vi "Check ToStim Queue.vi"(8 "error in (no error)":errorcluster, 11 "Stim Player Data In":T1) -> (0 "error out":errorcluster, 3 "Stim Player Data Out":T1, 4 "Error?":bool)   [LabVIEW 2011]
uses:
  Controls/Stim Player Data.ctl
  Controls/Top Level Control.ctl
  <vilib>/NI/AMC/Message Queue.ctl
  <vilib>/NI/AMC/Message.ctl
  <vilib>/NI/Tools/Keyed Array/KeyedArray.ctl
  Controls/ListBox Test Record.ctl
  Controls/DVR of CSV Tests Data.ctl
  Controls/CSVs Tests Data.ctl
  Controls/Test Column Data.ctl
  Controls/Options DVR.ctl
  Controls/Options.ctl
  <vilib>/NI Veristand/Execution/Workspace/WorkspaceAPI.ctl
  NationalInstruments.VeriStand.ClientAPI
  <vilib>/NI Veristand/Execution/SequenceExecutionInterface/Stimulus Profile Session Ref.ctl
  <vilib>/NI Veristand/Execution/ChannelFaultManager/ChannelFaultAPI.ctl
  <vilib>/NI/AMC/Create Single Message.vi
  <vilib>/NI/AMC/Update Message Routing Info.vi
  <vilib>/NI/AMC/Read Termination Message.vi
  <vilib>/NI/AMC/Globals.vi
  <vilib>/NI/AMC/Send Message.vi
  <vilib>/NI Veristand/Execution/SequenceExecutionInterface/NI_VS Sequence Execution Interface.lvlib
  <vilib>/NI/AMC/AMC.lvlib
  <vilib>/NI/Tools/Keyed Array/Tools_KeyedArray.lvlib
  <vilib>/NI Veristand/Execution/Workspace/NI_VS Workspace ExecutionAPI.lvlib
  <vilib>/NI Veristand/Execution/ChannelFaultManager/NI_VS ChannelFault ExecutionAPI.lvlib
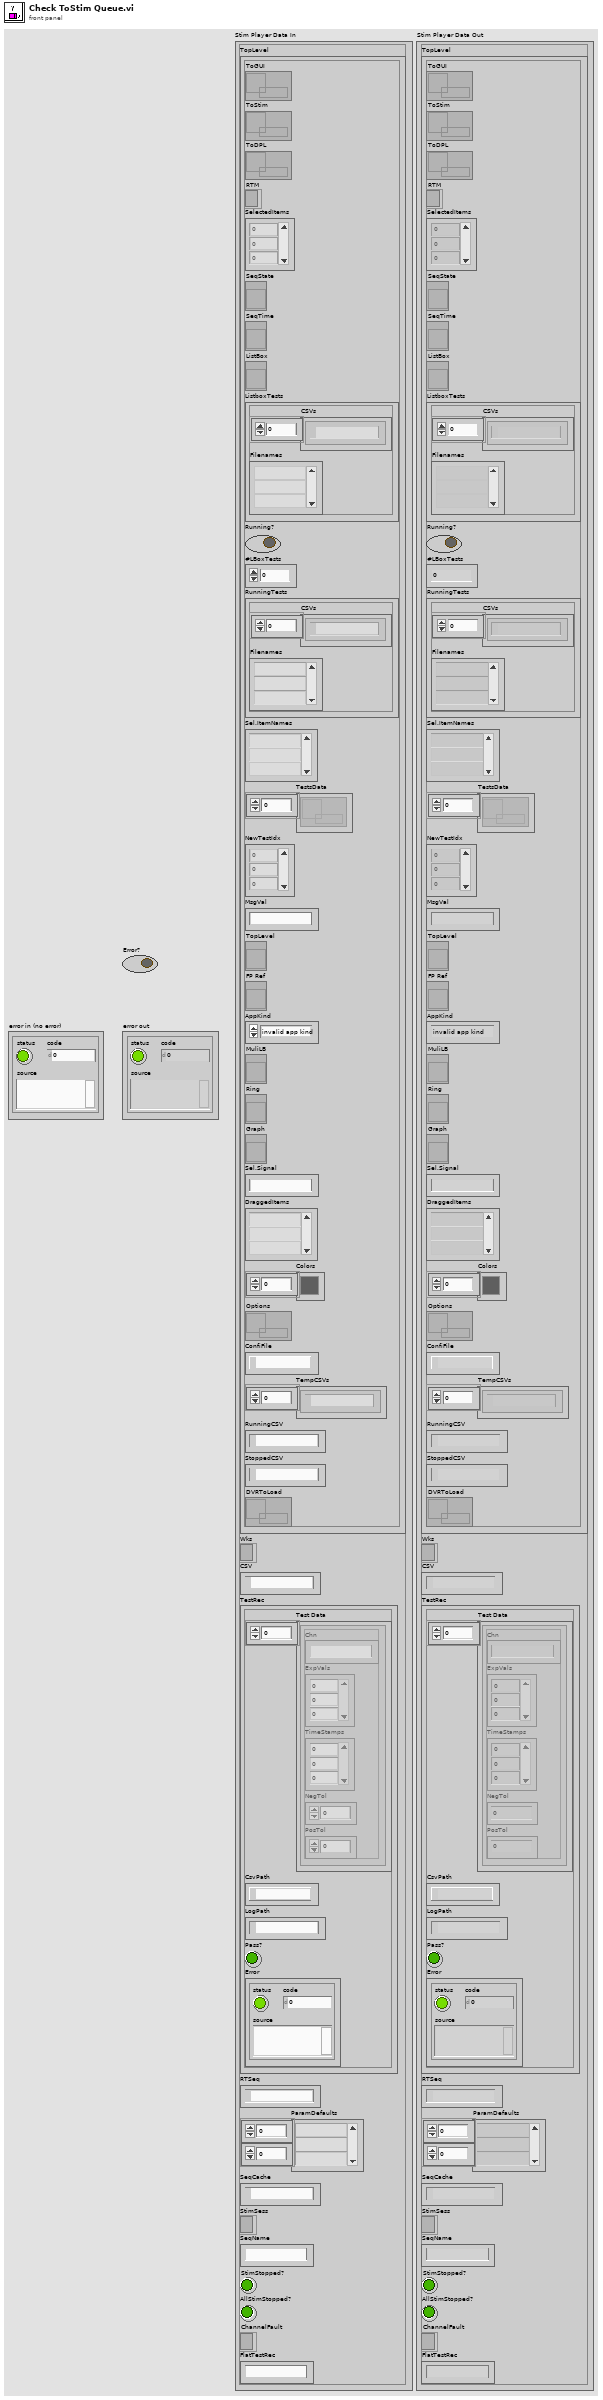
[diagram p1: front panel]
types:
  T1 = typedef "Stim Player Data.ctl" = cluster{"TopLevel":T2, "Wks":T7, "CSV":path, "TestRec":T8, "RTSeq":path, "ParamDefaults":string[][], "SeqCache":path, "StimSess":T10, "SeqName":string, "StimStopped?":bool, "AllStimStopped?":bool, "ChannelFault":T11, "FlatTestRec":string}
  T2 = typedef "Top Level Control.ctl" = cluster{"ToGUI":T3, "ToStim":T3, "ToDPL":T3, "RTM":refnum<k9>, "SelectedItems":i32[], "SeqState":refnum<vi>, "SeqTime":refnum<vi>, "ListBox":refnum<vi>, "ListboxTests":T4, "Running?":bool, "#LBoxTests":i32, "RunningTests":T4, "Sel.ItemNames":string[], "TestsData":T5[], "NewTestIdx":i32[], "MsgVal":string, "TopLevel":refnum<vi>, "FP Ref":refnum<vi>, "AppKind":enum32{"invalid app kind", "Development System", "Run Time System", "Student Edition", "Embedded LabVIEW", "Evaluation", "Custom"}, "MuliLB":refnum<vi>, "Ring":refnum<vi>, "Graph":refnum<vi>, "Sel.Signal":string, "DraggedItems":string[], "Colors":u32[], "Options":T6, "ConfiFile":path, "TempCSVs":path[], "RunningCSV":path, "StoppedCSV":path, "DVRToLoad":T5}
  T3 = typedef "AMC.lvlib/Message Queue.ctl" = refnum<queue>
  T4 = typedef "ListBox Test Record.ctl" = cluster{"CSVs":path[], "Filenames":string[]}
  T5 = typedef "DVR of CSV Tests Data.ctl" = refnum<data-value>
  T6 = typedef "Options DVR.ctl" = refnum<data-value>
  T7 = typedef "NI_VS Workspace ExecutionAPI.lvlib/WorkspaceAPI.ctl" = refnum<k24>
  T8 = typedef "CSVs Tests Data.ctl" = cluster{"Test Data":T9[], "CsvPath":path, "LogPath":path, "Pass?":bool, "Error":errorcluster}
  T9 = typedef "Test Column Data.ctl" = cluster{"Chn":string, "ExpVals":dbl[], "TimeStamps":i64[], "NegTol":dbl, "PosTol":dbl}
  T10 = typedef "NI_VS Sequence Execution Interface.lvlib/Stimulus Profile Session Ref.ctl" = refnum<k24>
  T11 = typedef "NI_VS ChannelFault ExecutionAPI.lvlib/ChannelFaultAPI.ctl" = refnum<k24>
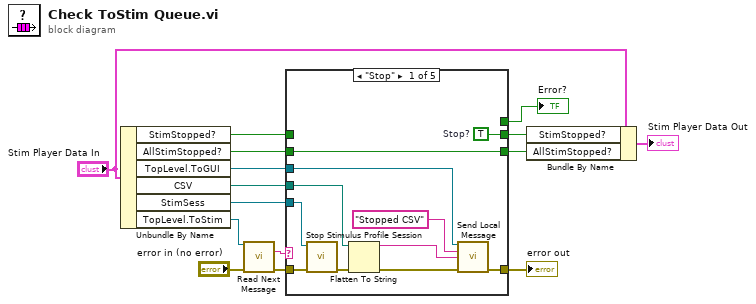
[diagram p0: block diagram]
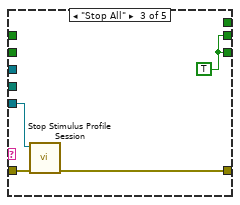
[diagram p3: hidden frame]
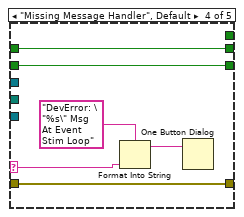
[diagram p4: hidden frame]
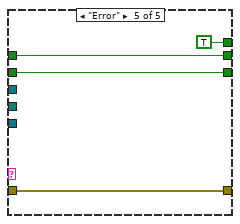
[diagram p5: hidden frame]
diagram:
  n1 = Unbundle By Name("Stim Player Data In") -> ("StimStopped?"=w10:bool, "AllStimStopped?"=w9:bool, "TopLevel.ToGUI"=w2:T3, "CSV"=w1:path, "StimSess"=w3:T10, "TopLevel.ToStim"=w4:T3)
  n2 = call <vilib>:"Read Next Message.vi"("message queue in"=w4, "error in"="error in (no error)") -> ("message name"=w11:string, "error out"=w12:errorcluster)  [unwired: 6 in, 6 out]
  n3 = case shown="\"Stop\"" w11 {
    selector: w11 -> [_ _ _ w37 _]
    tunnel: w12 -> [w26 w29 w33 w36 w43]
    tunnel: [w25 w29 w32 w36 w43] -> w14
    tunnel: [_ _ _ _ TRUE] -> w15
    tunnel: w9 -> [w20 w28 _ w35 w42]
    tunnel: [w20 w28 w31 w35 w42] -> w5
    tunnel: w10 -> [_ w27 _ w34 w40]
    tunnel: [w19 w27 w31 w34 w40] -> w6
    tunnel: w3 -> [w18 _ w30 _ _]
    tunnel: w2 -> [w17 _ _ _ _]
    tunnel: w1 -> [w16 _ _ _ _]
    frame "Stop" {
      w19 = TRUE  # Stop?
      n4 = call <vilib>:"Stop Stimulus Profile Session.vi"("error in (no error)"=w26, "Session Ref in"=w18) -> ("error out"=w24:errorcluster)  [unwired: 8 in, 1 out]
      n5 = Flatten To String(anything=w16, error in (no error)=w24) -> (data string=w22:string, error out=w21:errorcluster)  [unwired: 2 in, 1 out]
      n6 = call <vilib>:"Send Local Message.vi"("message queue in"=w17, "message name"="Stopped CSV" ("Message Name"), "message value"=w22, "error in"=w21) -> ("error out"=w25:errorcluster)  [unwired: 9 in, 2 out]
    }
    frame "" {
    }
    frame "Stop All" {
      w31 = TRUE
      n7 = call <vilib>:"Stop Stimulus Profile Session.vi"("error in (no error)"=w33, "Session Ref in"=w30) -> ("error out"=w32:errorcluster)  [unwired: 8 in, 1 out]
    }
    frame "Missing Message Handler", Default {
      n8 = Format Into String(format string="DevError: \"%s\" Msg At Event Stim Loop" ("message"), w37) -> (resulting string=w39:string)  [unwired: 2 in, 1 out]
      n9 = One Button Dialog(message=w39) -> ()  [unwired: 2 out]
    }
    frame "Error" {
    }
  }
  "Error?" <- w15
  "error out" <- w14
  n10 = Bundle By Name(cluster="Stim Player Data In", "StimStopped?"=w6, "AllStimStopped?"=w5) -> (→"Stim Player Data Out":T1)
